vi "Receive Tree Double Click.vi"(8 "error in (no error)":errorcluster, 10 "TreeDoubleClickMsg":refnum<class "TreeDoubleClickMsg.lvclass">, 11 "IEventAggregator In":refnum<class "IEventAggregator.lvclass">) -> (0 "error out":errorcluster, 3 "IEventAggregator Out":refnum<class "IEventAggregator.lvclass">)   [LabVIEW 2020, in "ActorEvents.lvlib" / "IEventAggregator.lvclass"]
doc: "<License>\nCopyright © 2017 Composed Systems, LLC | All rights reserved\nwww.composed.io\n\nAuthor: Ethan Stern <ethan.stern@composed.io>\n\nThis software is provided \"AS IS\" WITHOUT WARRANTIES, either express or implied, AND IS FOR EDUCATIONAL PURPOSES ONLY.\n</License>"
uses:
  <vilib>/gpm_packages/@cs/mva-viewable/Source/ActorEvents/IEventAggregator/IEventAggregator.lvclass
  <vilib>/gpm_packages/@cs/mva-viewable/Source/ActorEvents/IEventAggregator Messages/TreeDoubleClickMsg/TreeDoubleClickMsg.lvclass
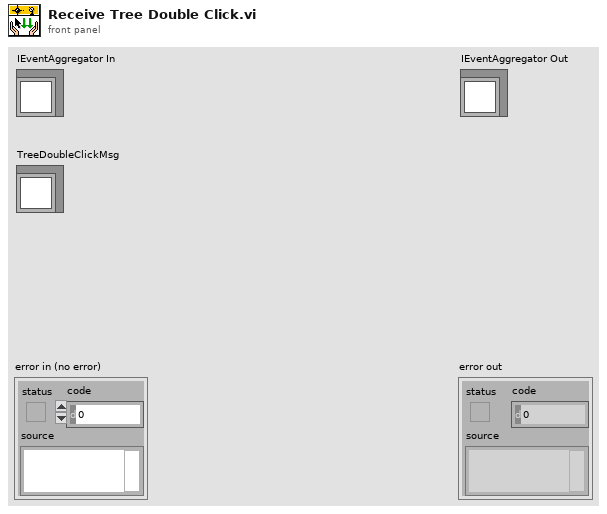
[diagram p1: front panel]
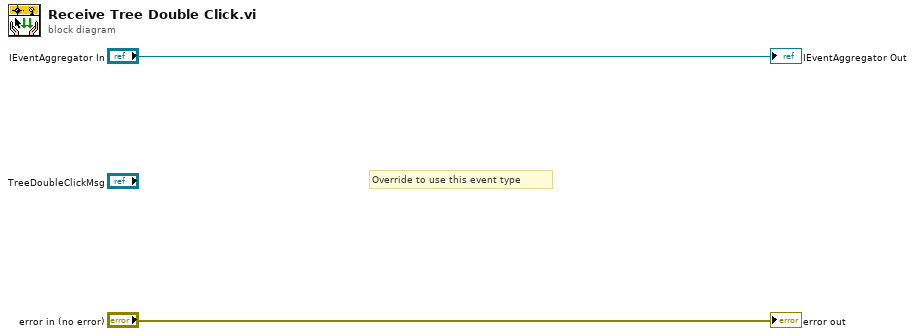
[diagram p0: block diagram]
diagram:
  # "Override to use this event type"
  "error out" <- "error in (no error)"
  "IEventAggregator Out" <- "IEventAggregator In"
